vi "Read Configuration Parameters.vi"(8 "error in (no error)":errorcluster, 10 "refnum":T1, 11 "Example Configuration Dialog in":refnum<class "Example Configuration Dialog.lvclass">) -> (0 "error out":errorcluster, 2 "refnum out":T1, 3 "Example Configuration Dialog out":refnum<class "Example Configuration Dialog.lvclass">)   [LabVIEW 2017, in "Example Configuration Dialog.lvlib" / "Example Configuration Dialog.lvclass"]
uses:
  Example Configuration Dialog.lvclass
  <vilib>/Utility/config.llb/Config Data RefNum.ctl
  Example Configuration Dialog.lvclass/Example Configuration Dialog.ctl
  <vilib>/Utility/config.llb/Read Key (I32).vi
  <vilib>/Utility/config.llb/Read Key (String).vi
  Configuration.lvclass
  <vilib>/Utility/config.llb/NI_LVConfig.lvlib
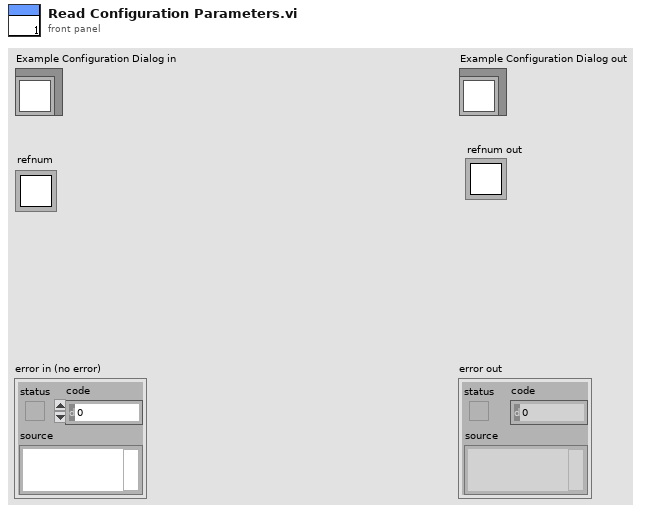
[diagram p1: front panel]
types:
  T1 = typedef "NI_LVConfig.lvlib/Config Data RefNum.ctl" = refnum<k1>
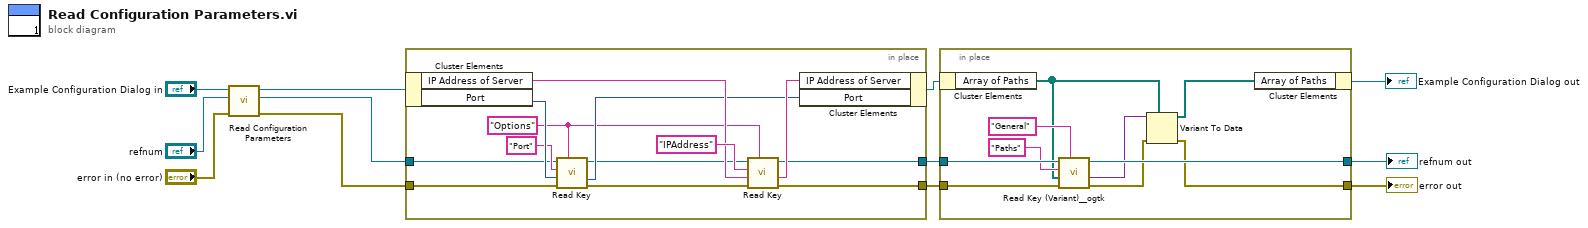
[diagram p0: block diagram]
diagram:
  n1 = call-parent "Read Configuration Parameters.vi"("error in (no error)"="error in (no error)", "refnum"="refnum", "Configuration in"="Example Configuration Dialog in") -> ("error out"=w8:errorcluster, "refnum out"=w9:T1, "Configuration out"=w7:refnum<class "Example Configuration Dialog.lvclass">)  [unwired: 6 in]
  n2 = in-place "In Place Element Structure" {
    in-place-border: w9 -> [w14]
    in-place-border: w8 -> [w20]
    in-place-border: [w22] -> w4
    in-place-border: [w21] -> w5
    w16 = "Options" ("section")
    n3 = in-place-cluster #1(w7) -> ("IP Address of Server"=w23:string, "Port"=w18:i32)
    n4 = call-poly <vilib>:"Read Key.vi"("section"=w16, "error in (no error)"=w20, "default value"=w18, "key"="Port", "refnum"=w14) -> ("error out"=w19:errorcluster, "value"=w17:i32, "refnum out"=w13:T1)  [unwired: 3 in, 1 out]
    n5 = call-poly <vilib>:"Read Key.vi"("section"=w16, "error in (no error)"=w19, "default value"=w23, "key"="IPAddress", "refnum"=w13) -> ("error out"=w22:errorcluster, "value"=w24:string, "refnum out"=w21:T1)  [unwired: 3 in, 1 out]
    n6 = in-place-cluster #1("IP Address of Server"=w24, "Port"=w17) -> (w6:refnum<class "Example Configuration Dialog.lvclass">)
  }
  n7 = in-place "In Place Element Structure" {
    in-place-border: w5 -> [w35]
    in-place-border: w4 -> [w34]
    in-place-border: [w26] -> w3
    in-place-border: [w31] -> w2
    n8 = in-place-cluster #2(w6) -> ("Array of Paths"=w30:path[])
    n9 = call <userlib>:"Read Key (Variant)__ogtk.vi"("section"="General", "error in (no error)"=w34, "type"=w30, "key (optional)"="Paths", "refnum"=w35) -> ("error out"=w27:errorcluster, "key-value"=w29:variant, "refnum out"=w31:T1)  [unwired: 3 in, 1 out]
    n10 = Variant To Data(error in=w27, type=w30, Variant=w29) -> (data=w28:path[], error out=w26:errorcluster)
    n11 = in-place-cluster #2("Array of Paths"=w28) -> (→"Example Configuration Dialog out":refnum<class "Example Configuration Dialog.lvclass">)
  }
  "error out" <- w3
  "refnum out" <- w2
